vi "Save_Cluster_to_Spreadsheet.vi"() -> ()   [LabVIEW 2025]
panel:
  in  "stop":bool
  in  "Save":bool
  in  "Test Cluster":T1={"Date"="10-06-22", "Test Name"="Power Consumption Test", "Serial Number"="APCK7895DS", "Operator Name"="Michael Malone"}
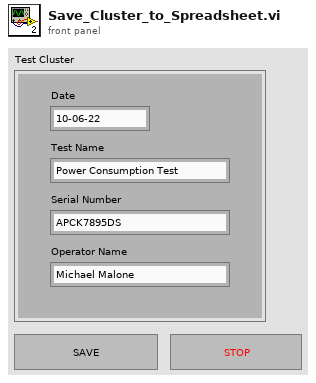
[diagram p1: front panel]
types:
  T1 = cluster{"Date":string, "Test Name":string, "Serial Number":string, "Operator Name":string}
  T2 = cluster{"Date":string, "Test Name":string, "Result":string, "Operator Name":string}
  T3 = enum16{"open", "replace", "create", "open or create", "replace or create", "replace or create with confirmation"}
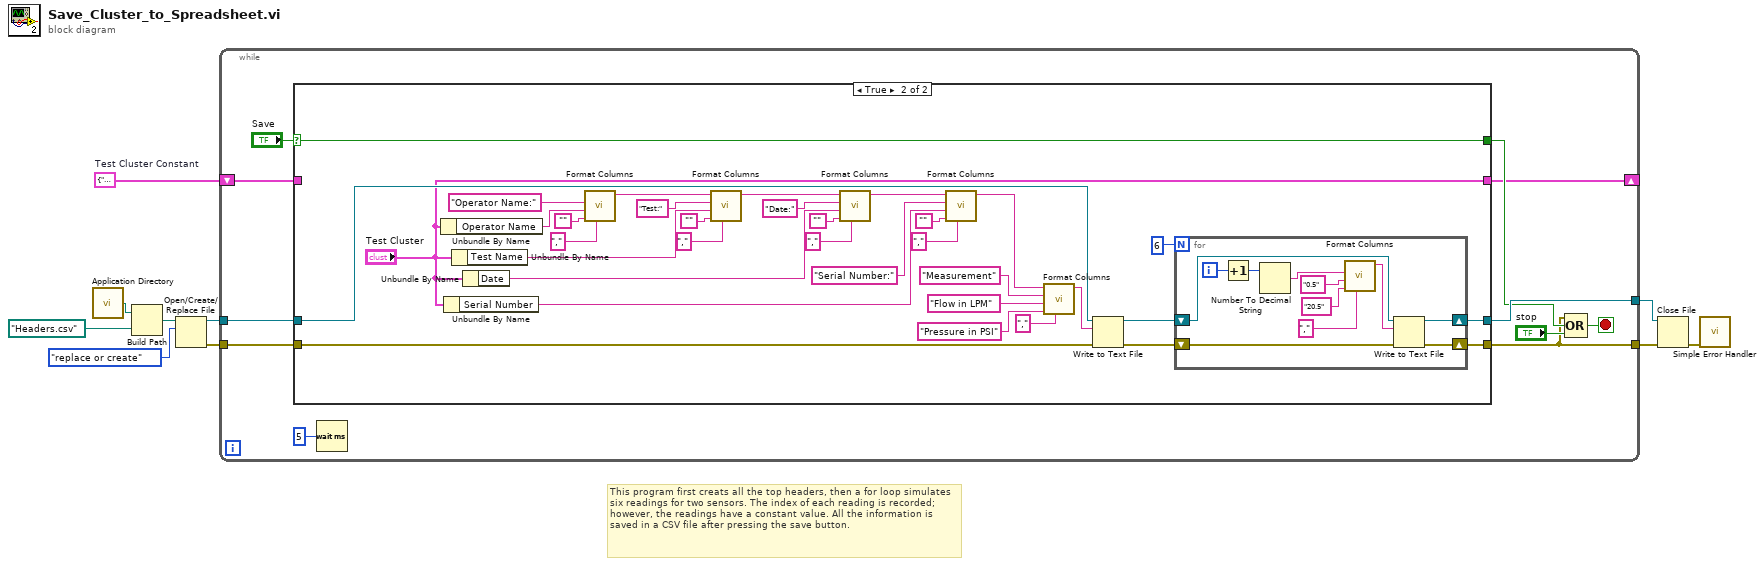
[diagram p0: block diagram]
diagram:
  w3 = T2 {"Date"="", "Test Name"="", "Result"="", "Operator Name"=""}  # Test Cluster Constant
  # "This program first creats all the top headers, then a for loop simulates six readings for two sensors. The index of each reading is recorded; however, the readings have a constant value. All the information is saved in a CSV file after pressing the save button."
  n1 = call <vilib>:"Application Directory.vi"() -> ("Application Directory"=w10:path)
  n2 = Build Path(base path=w10, name or relative path=path "Headers.csv") -> (appended path=w8:path)
  n3 = Open/Create/Replace File(file path (use dialog)=w8, operation (0:open)=T3."replace or create") -> (refnum out=w6:refnum<file>, error out=w5:errorcluster)  [unwired: 4 in, 1 out]
  n4 = while {
    tunnel: w6 -> [w20]
    tunnel: w5 -> [w19]
    shift-right: [w11] -> _
    shift-left: w3 -> [w17]
    tunnel: [w13] -> w2
    tunnel: [w16] -> w1
    stop <- w12 stop-if-true
    n5 = case shown="True" "Save" {
      selector: "Save" -> [_ w56]
      tunnel: w20 -> [w23 w58]
      tunnel: w19 -> [w22 w57]
      tunnel: [w22 w27] -> w13
      tunnel: [w23 w25] -> w16
      tunnel: [w24 "Test Cluster"] -> w11
      tunnel: w17 -> [w24 _]
      tunnel: [_ w56] -> w14
      frame False {
      }
      frame True {
        n6 = Unbundle By Name("Test Cluster") -> ("Operator Name"=w54:string)
        n7 = Unbundle By Name("Test Cluster") -> ("Serial Number"=w37:string)
        n8 = Unbundle By Name("Test Cluster") -> ("Test Name"=w49:string)
        n9 = Unbundle By Name("Test Cluster") -> ("Date"=w45:string)
        n10 = call "Format Columns.vi"("Delimiter"=",", "Column 3"="", "Column 2"=w54, "Column 1"="Operator Name:") -> ("Result String"=w47:string)  [unwired: 7 in]
        n11 = call "Format Columns.vi"("Delimiter"=",", "Column 3"="", "Column 2"=w49, "Column 1"="Test:", "Last String"=w47) -> ("Result String"=w42:string)  [unwired: 6 in]
        n12 = call "Format Columns.vi"("Delimiter"=",", "Column 3"="", "Column 2"=w45, "Column 1"="Date:", "Last String"=w42) -> ("Result String"=w36:string)  [unwired: 6 in]
        n13 = call "Format Columns.vi"("Delimiter"=",", "Column 3"="", "Column 2"=w37, "Column 1"="Serial Number:", "Last String"=w36) -> ("Result String"=w35:string)  [unwired: 6 in]
        n14 = call "Format Columns.vi"("Delimiter"=",", "Column 3"="Pressure in PSI", "Column 2"="Flow in LPM", "Column 1"="Measurement", "Last String"=w35) -> ("Result String"=w30:string)  [unwired: 6 in]
        n15 = Write to Text File(file (use dialog)=w58, text=w30, error in=w57) -> (refnum out=w26:refnum<file>, error out=w28:errorcluster)  [unwired: 1 in, 1 out]
        n16 = for {
          N: 6 -> [_]
          shift-right: [w60] -> w25
          shift-left: w26 -> [w61]
          shift-right: [w62] -> w27
          shift-left: w28 -> [w63]
          i -> [w69]
          n17 = Increment(x=w69) -> (x+1=w68:i32)
          n18 = Number To Decimal String(number=w68) -> (decimal integer string=w67:string)  [unwired: 1 in]
          n19 = call "Format Columns.vi"("Delimiter"=",", "Column 3"="20.5", "Column 2"="0.5", "Column 1"=w67) -> ("Result String"=w59:string)  [unwired: 7 in]
          n20 = Write to Text File(file (use dialog)=w61, text=w59, error in=w63) -> (refnum out=w60:refnum<file>, error out=w62:errorcluster)  [unwired: 1 in, 1 out]
        }
      }
    }
    n21 = Wait (ms)(milliseconds to wait=u32 5) -> ()  [unwired: 1 out]
    n22 = Compound Arithmetic op=OR(w13, w14, "stop") -> (w12:bool)
  }
  n23 = Close File(refnum=w1, error in=w2) -> (error out=w4:errorcluster)  [unwired: 1 out]
  n24 = call <vilib>:"Simple Error Handler.vi"("error in (no error)"=w4) -> ()  [unwired: 4 in, 5 out]
